vi "CreateMeanderMask_3d.vi"(7 "Rep. Rate (Hz)":dbl=10.0 min=0.0 max=34.0, 10 "Start Position":dbl[](array[numeric]) min=0.0 max=34.0) -> (0 "Laser_Ctrl":bool, 1 "start/end points":cluster{dbl, dbl, dbl}[][](array[cluster]), 2 "Canceled":bool, 5 "ImageParameter":T1)   [LabVIEW 2013]
uses:
  ImagingMS/ImageConvPara.ctl
panel:
  in  "Apply":bool
  in  "X StepWidth":dbl=0.05 min=0.0 max=34.0
  in  "Imaging?":bool
  out "Estimated Time (min)":dbl min=0.0 max=34.0
  in  "Average/pixel":i32=10 min=0 max=34
  in  "Cancel":bool
  in  "Run":bool
  out "XY Graph":cluster{dbl, dbl, "X StepWidth":dbl}[](graph)
  out "Y Size (mm)":dbl min=0.0 max=34.0
  out "X Size (mm)":dbl min=0.0 max=34.0
  in  "Y Steps":i32=50 min=0 max=34
  in  "X Size":dbl=2.0 min=0.0 max=34.0
  in  "Y StepWidth":dbl=0.05 min=0.0 max=34.0
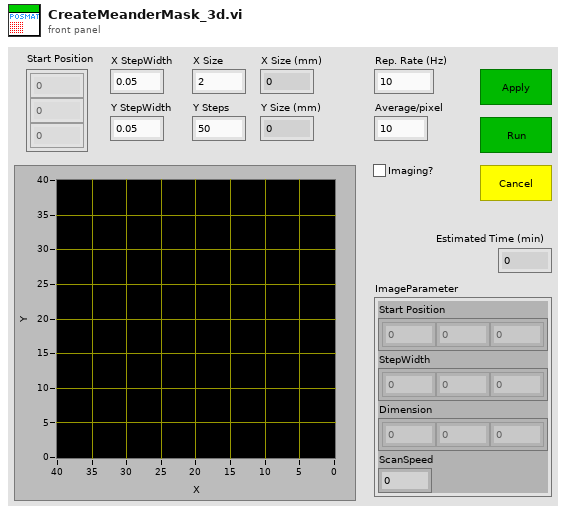
[diagram p1: front panel]
types:
  T1 = typedef "ImageConvPara.ctl" = cluster{"Start Position":dbl[], "StepWidth":dbl[], "Dimension":i32[], "ScanSpeed":dbl}
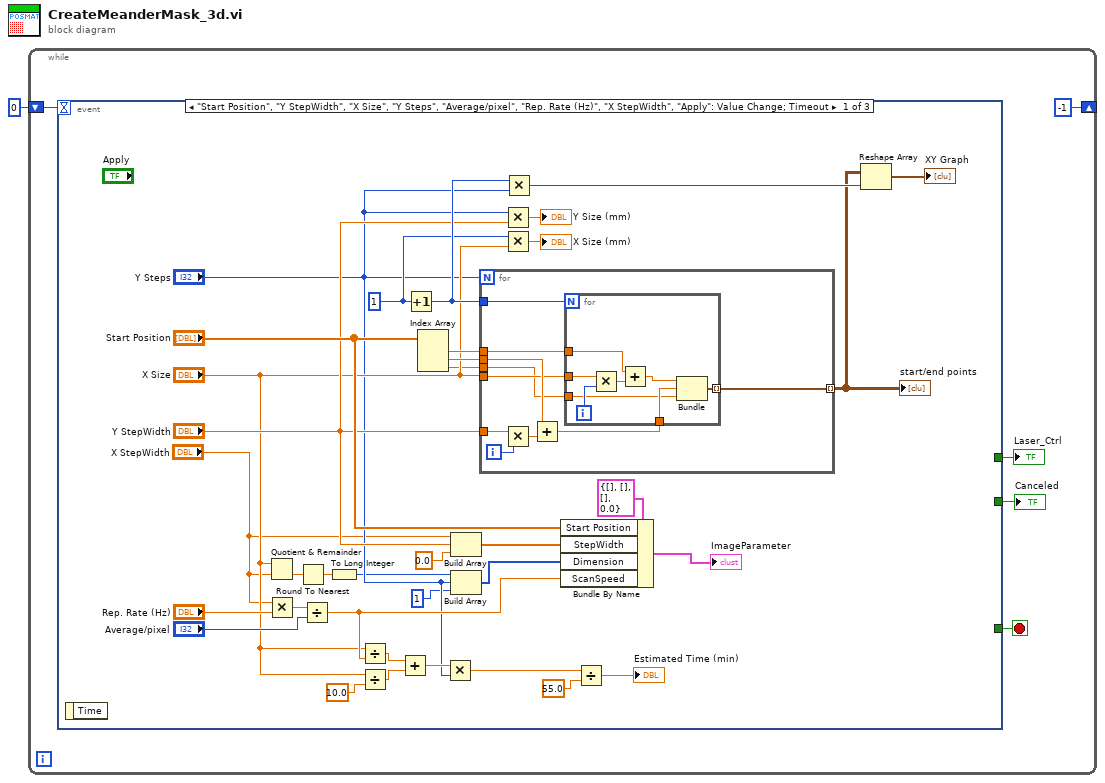
[diagram p0: block diagram]
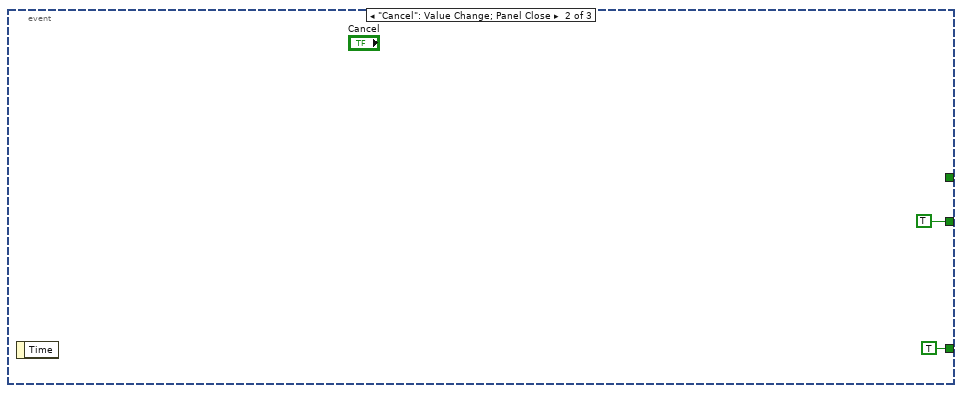
[diagram p2: hidden frame]
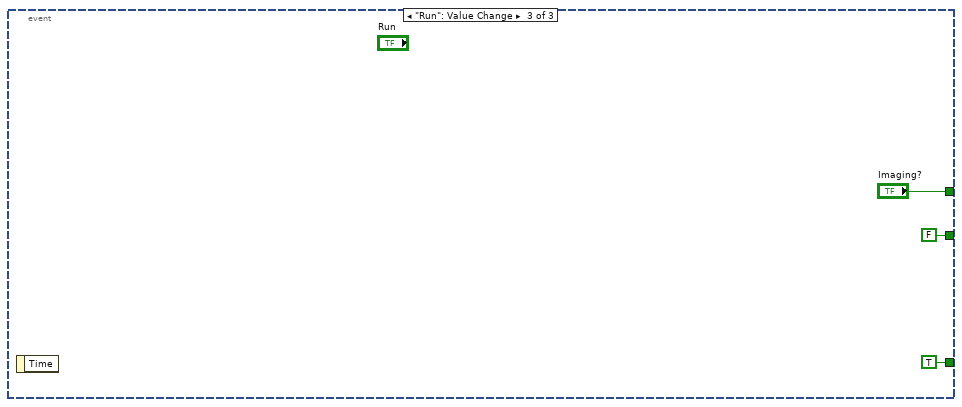
[diagram p3: hidden frame]
diagram:
  n1 = while {
    shift-right: [-1] -> _
    shift-left: 0 -> [w3]
    stop <- w6 stop-if-true
    n2 = event shown="[0] \"Start Position\", \"Y StepWidth\", \"X Size\", \"Y Steps\", \"Average/pixel\", \"Rep. Rate (Hz)\", \"X StepWidth\", \"Apply\": Value Change;  Timeout" {
      selector: _ -> [_ _ _]
      dyn-events: _ -> [_ _ _]
      timeout: w3 -> [_ _ _]
      tunnel: [_ TRUE TRUE] -> w6
      tunnel: [_ TRUE ("Canceled") FALSE ("Canceled")] -> w5
      tunnel: [_ _ "Imaging?"] -> w4
      event "Start Position", "Y StepWidth", "X Size", "Y Steps", "Average/pixel", "Rep. Rate (Hz)", "X StepWidth", "Apply": Value Change; Timeout {
        w35 = 1
        n3 = event-data() -> ()  [unwired: 1 in, 1 out]
        n4 = Quotient & Remainder(x="X Size", y="X StepWidth") -> (floor(x/y)=w27:dbl)  [unwired: 1 out]
        n5 = Multiply(x="X StepWidth", y="Rep. Rate (Hz)") -> (x*y=w26:dbl)
        n6 = Round To Nearest(number=w27) -> (nearest integer value=w10:dbl)
        n7 = Divide(x=w26, y="Average/pixel") -> (x/y=w22:dbl)
        n8 = To Long Integer(number=w10) -> (32bit integer=w11:i32)
        n9 = Divide(x="X Size", y=w22) -> (x/y=w20:dbl)
        n10 = Divide(x="X Size", y=10.0) -> (x/y=w19:dbl)
        n11 = Add(x=w20, y=w19) -> (x+y=w18:dbl)
        n12 = Increment(x=w35) -> (x+1=w36:i32)
        n13 = Index Array(array="Start Position") -> (element #1=w41:dbl, element #2=w40:dbl, element #3=w13:dbl)  [unwired: 3 in]
        n14 = Multiply(x=w18, y="Y Steps") -> (x*y=w17:dbl)
        n15 = Build Array("X StepWidth", "Y StepWidth", 0.0 ("element")) -> (w30:dbl[])
        n16 = Build Array(w11, "Y Steps", 1 ("element")) -> (w29:i32[])
        n17 = for {
          N: "Y Steps" -> [_]
          tunnel: w40 -> [w46]
          tunnel: "Y StepWidth" -> [w42]
          tunnel: "X Size" -> [w45]
          tunnel: w36 -> [w48]
          tunnel: [w47] -> w33 mode=indexing
          tunnel: w13 -> [w43]
          tunnel: w41 -> [w44]
          i -> [w51]
          n18 = Multiply(x=w42, y=w51) -> (x*y=w50:dbl)
          n19 = Add(x=w46, y=w50) -> (x+y=w49:dbl)
          n20 = for {
            N: w48 -> [_]
            tunnel: w45 -> [w57]
            tunnel: w44 -> [w52]
            tunnel: w49 -> [w55]
            tunnel: [w56] -> w47 mode=indexing
            tunnel: w43 -> [w53]
            i -> [w58]
            n21 = Multiply(x=w57, y=w58) -> (x*y=w59:dbl)
            n22 = Add(x=w52, y=w59) -> (x+y=w54:dbl)
            n23 = Bundle(w54, w55, "X StepWidth"=w53) -> (w56:cluster{dbl, dbl, "X StepWidth":dbl})  [unwired: 1 in]
          }
        }
        "start/end points" <- w33
        n24 = Multiply(x="Y Steps", y="Y StepWidth") -> (x*y=→"Y Size (mm)":dbl)
        n25 = Multiply(x=w35, y="X Size") -> (x*y=→"X Size (mm)":dbl)
        n26 = Multiply(x=w36, y="Y Steps") -> (x*y=w37:i32)
        n27 = Bundle By Name(cluster=T1 {"Start Position"=[], "StepWidth"=[], "Dimension"=[], "ScanSpeed"=0.0} ("ImageParameter"), "Start Position"="Start Position", "StepWidth"=w30, "Dimension"=w29, "ScanSpeed"=w22) -> (→"ImageParameter":T1)
        n28 = Divide(x=w17, y=55.0) -> (x/y=→"Estimated Time (min)":dbl)
        n29 = Reshape Array(w33, w37) -> (→"XY Graph":cluster{dbl, dbl, "X StepWidth":dbl}[])
      }
      event "Cancel": Value Change; Panel Close {
        n30 = event-data() -> ()  [unwired: 1 in, 1 out]
      }
      event "Run": Value Change {
        n31 = event-data() -> ()  [unwired: 1 in, 1 out]
      }
    }
    "Canceled" <- w5
    "Laser_Ctrl" <- w4
  }
